vi "Broadcast Diverter Port.vi"(8 "error in (no error)":errorcluster, 10 "Reply Payload":T1) -> (0 "error out":errorcluster)   [LabVIEW 2020, in "Spectrometer.lvlib"]
doc: "_____\nCreated using Delacor QMH Event Scripter 5.0.0.112."
uses:
  Spectrometer.lvlib
  Set Diverter Port (Reply Payload)--cluster.ctl
  SpectraPro-LabVIEW-Driver/Libraries/Types/Diverter Port.ctl
  SpectraPro-LabVIEW-Driver/SpectraPro.lvlib
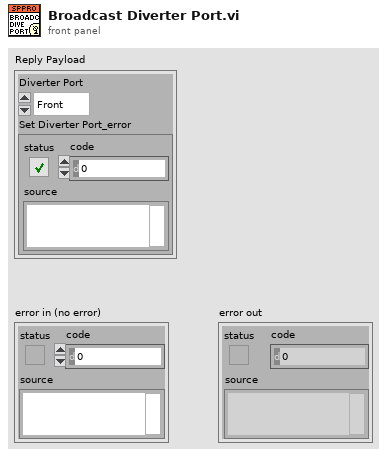
[diagram p1: front panel]
types:
  T1 = typedef "Spectrometer.lvlib/Set Diverter Port (Reply Payload)--cluster.ctl" = cluster{"Diverter Port":T2, "Set Diverter Port_error":errorcluster}
  T2 = typedef "SpectraPro.lvlib/Diverter Port.ctl" = enum16{"Front", "Side"}
  T3 = typedef "Spectrometer.lvlib/Broadcast Events--cluster.ctl" = cluster{"Module Did Init":refnum<user-event>, "Status Updated":refnum<user-event>, "Error Reported":refnum<user-event>, "Module Did Stop":refnum<user-event>, "Update Module Execution Status":refnum<user-event>, "Broadcast Wavelength":refnum<user-event>, "Broadcast Slit Width":refnum<user-event>, "Broadcast Grating":refnum<user-event>, "Broadcast Diverter Port":refnum<user-event>}
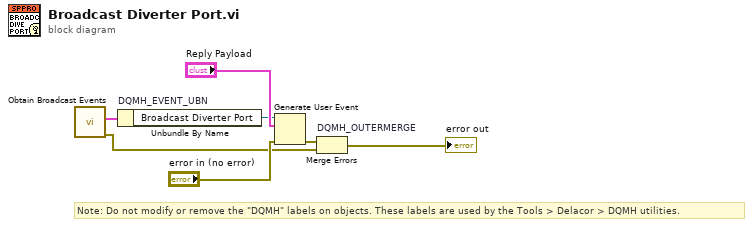
[diagram p0: block diagram]
diagram:
  # "Note: Do not modify or remove the \"DQMH\" labels on objects. These labels are used by the Tools > Delacor > DQMH utilities."
  n1 = call "Obtain Broadcast Events.vi"() -> ("error out"=w2:errorcluster, "Spectrometer Broadcast Events"=w1:T3)  [unwired: 10 in]
  n2 = Unbundle By Name "DQMH_EVENT_UBN"(w1) -> ("Broadcast Diverter Port"=w4:refnum<user-event>)
  n3 = Generate User Event(user event=w4, event data cluster="Reply Payload", error in="error in (no error)") -> (error out=w3:errorcluster)  [unwired: 1 in, 1 out]
  n4 = Merge Errors "DQMH_OUTERMERGE"(w3, w2) -> (→"error out":errorcluster)
